vi "CMD_Run.vi"(1 "Line":string) -> (0 "Done":bool)   [LabVIEW 2017, in "Apple script.lvlib"]
uses:
  Apple script.lvlib
  <vilib>/Rock Robotics/WPI/ThirdParty/Phoenix-LabVIEW/Motor Controller/Controls/CTRE_Phoenix_MotorControl_ControlMode.ctl
panel:
  in  "Parameters":i32[](array[numeric])=[1, 1, 1, 1]
  in  "Subcommands":string[](array[string])=["motor", "at", "for", "until"]
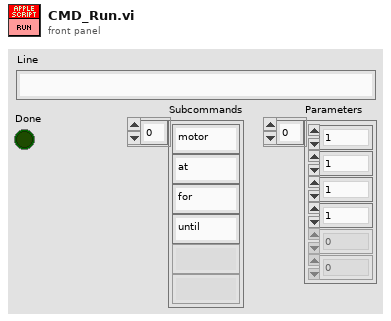
[diagram p1: front panel]
types:
  T1 = typedef "CTRE_Phoenix_MotorControl_ControlMode.ctl" = u16
  T2 = typedef "WPI_MotorControlDeviceRef.ctl" = cluster{"DeviceStatus":errorcluster, "Type":T3, "PWM":cluster{"PWM Channel":T4, "DeadBand":T5}, "CAN":cluster{"Device Number":u8, "SetOutput VI Ref":variant, "GetOutput VI Ref":variant, "Enable VI Ref":variant, "Disable VI Ref":variant, "Data":variant}, "Invert":bool, "DIO PWM":cluster{"PWM \"Enable\" Channel":T4, "DIOChannel":T6, "PWM Rate":dbl}}
  T3 = typedef "WPI_MotorControlType.ctl" = enum16{"PWM", "CAN", "DIO PWM"}
  T4 = typedef "FPGA_DIOPWMChannel.ctl" = enum8{"PWM 0", "PWM 1", "PWM 2", "PWM 3", "PWM 4", "PWM 5", "PWM 6", "PWM 7", "PWM 8", "PWM 9", "PWM MXP 0", "PWM MXP 1", "PWM MXP 2", "PWM MXP 3", "PWM MXP 4", "PWM MXP 5", "PWM MXP 6", "PWM MXP 7", "PWM MXP 8", "PWM MXP 9", "Invalid"}
  T5 = typedef "WPI_PWMDeadband.ctl" = cluster{"Name":string, "maxPositivePwm":i32, "minPositivePwm":i32, "centerPwm":i32, "maxNegativePwm":i32, "minNegativePwm":i32, "angularRange":u16}
  T6 = typedef "FPGA_DIOChannel.ctl" = enum8{"DIO 0", "DIO 1", "DIO 2", "DIO 3", "DIO 4", "DIO 5", "DIO 6", "DIO 7", "DIO 8", "DIO 9", "DIO MXP 0", "DIO MXP 1", "DIO MXP 2", "DIO MXP 3", "DIO MXP 4", "DIO MXP 5", "DIO MXP 6", "DIO MXP 7", "DIO MXP 8", "DIO MXP 9", "DIO MXP 10", "DIO MXP 11", "DIO MXP 12", "DIO MXP 13", "DIO MXP 14", "DIO MXP 15", "SPI Port CS1", "SPI Port CS2", "SPI Port CS3", "SPI Port MISO", "SPI Port MOSI", "Invalid"}
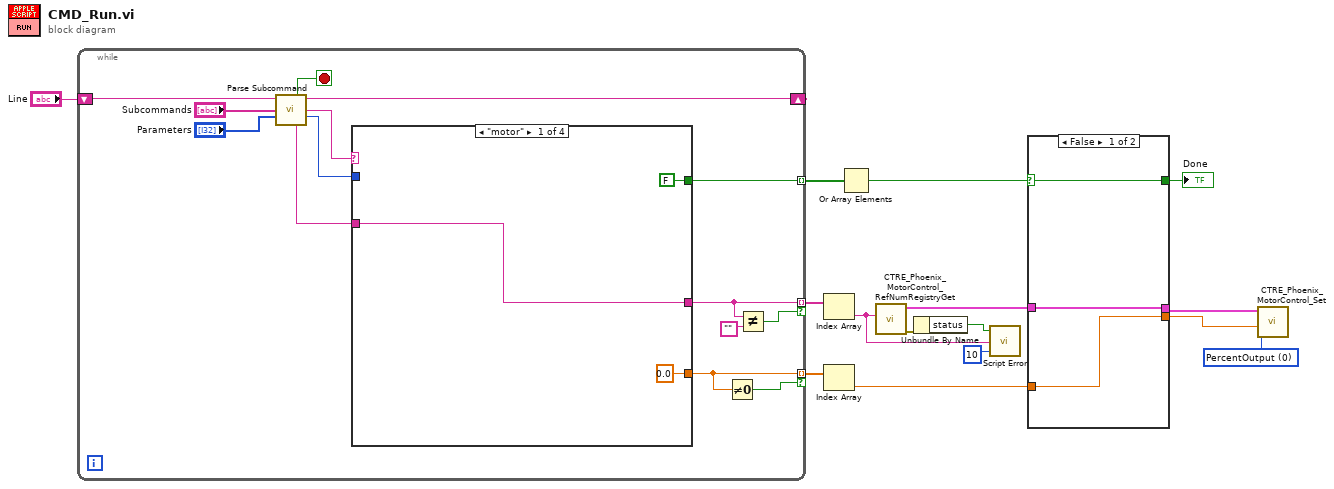
[diagram p0: block diagram]
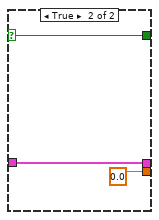
[diagram p2: hidden frame]
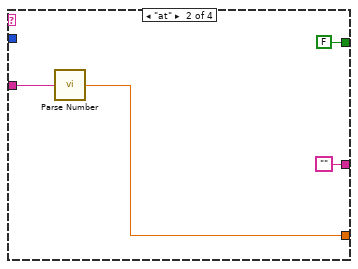
[diagram p3: hidden frame]
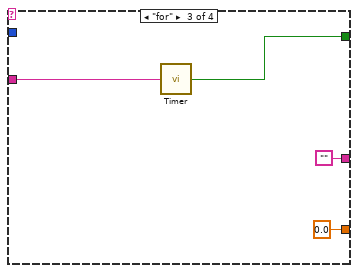
[diagram p4: hidden frame]
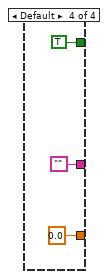
[diagram p5: hidden frame]
diagram:
  w5 = T1 0 items=["PercentOutput"=0, "Position"=1, "Velocity"=2, "Current"=3, "Follower"=5, "MotionProfile"=6, "MotionMagic"=7, "MotionMagicArc"=8, "MotionProfileArc"=10, "Disabled"=15] ("Control Mode")
  n1 = while {
    shift-right: [w26] -> _
    shift-left: "Line" -> [w29]
    tunnel: [w21] -> w14 mode=indexing
    tunnel: [w20] -> w13 mode=indexing if=w18
    tunnel: [w17] -> w12 mode=indexing if=w16
    stop <- w25 stop-if-true
    n2 = call "Parse Subcommand.vi"("Text In"=w29, "Subcommands"="Subcommands", "Parameters"="Parameters") -> ("Done"=w25:bool, "Text Out"=w26:string, "Subcommand"=w24:string, "# of Parameters"=w23:i32, "Parameter 1"=w22:string)  [unwired: 6 in, 2 out]
    n3 = case shown="\"motor\"" w24 {
      tunnel: w23 -> [_ _ _ _]
      tunnel: w22 -> [w30 w36 w40 _]
      tunnel: [FALSE FALSE ("Value") w37 TRUE ("Value")] -> w21
      tunnel: [w30 "" "" ""] -> w20
      tunnel: [0.0 ("Number") w33 0.0 ("Number") 0.0 ("Number")] -> w17
      frame "motor" {
      }
      frame "at" {
        n4 = call "Parse Number.vi"("String"=w36) -> ("Number"=w33:dbl)
      }
      frame "for" {
        n5 = call "Timer.vi"("Seconds (string)"=w40) -> ("Done"=w37:bool)
      }
      frame Default {
      }
    }
    n6 = Not Equal To 0?(x=w17) -> (x != 0?=w16:bool)
    n7 = Not Equal?(x=w20, y="") -> (x != y?=w18:bool)
  }
  n8 = Index Array(array=w13) -> (element=w3:string)  [unwired: 1 in]
  n9 = Index Array(array=w12) -> (element=w9:dbl)  [unwired: 1 in]
  n10 = Or Array Elements(Boolean array=w14) -> (logical OR=w11:bool)
  n11 = call <vilib>:"CTRE_Phoenix_MotorControl_RefNumRegistryGet.vi"("refnum name"=w3) -> ("error out"=w2:errorcluster, "PhoenixMotorControlDevRef"=w4:T2)  [unwired: 9 in]
  n12 = Unbundle By Name(w2) -> ("status"=w1:bool)
  n13 = call "Script Error.vi"("Error?"=w1, "Error Details"=w3, "Error Code"=10) -> ()  [unwired: 2 in, 1 out]
  n14 = case shown="False" w11 {
    selector: w11 -> [w46 w49]
    tunnel: [w46 w49] -> w10
    tunnel: w4 -> [w45 w48]
    tunnel: [w45 w48] -> w7
    tunnel: w9 -> [w44 _]
    tunnel: [w44 0.0] -> w6
    frame False {
    }
    frame True {
    }
  }
  "Done" <- w10
  n15 = call <vilib>:"CTRE_Phoenix_MotorControl_Set.vi"("Output"=w6, "Control Mode"=w5, "PhoenixMotorControlDevRef"=w7) -> ()  [unwired: 7 in, 2 out]
